vi "TagDB Refmgr-Register.vi"(7 "menu reference":refnum<k9>, 8 "error in (no error)":errorcluster, 9 "ViName":string, 10 "VI Refnum":refnum<vi>, 11 "TagDB in":refnum<k1>) -> (0 "error out":errorcluster, 2 "VI Refnum (dup)":refnum<vi>, 3 "TagDB out":refnum<k1>)   [LabVIEW 2017, in "TagDB RefManager.lvlib"]
uses:
  TagDB RefManager.lvlib
  _Support/Refnum Operation/VI/VIName.vi
  _Support/Refnum Operation/VI/Caller's VI Reference.vi
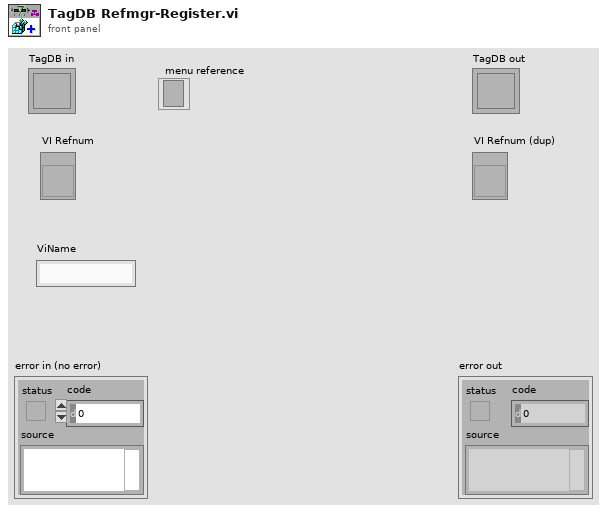
[diagram p1: front panel]
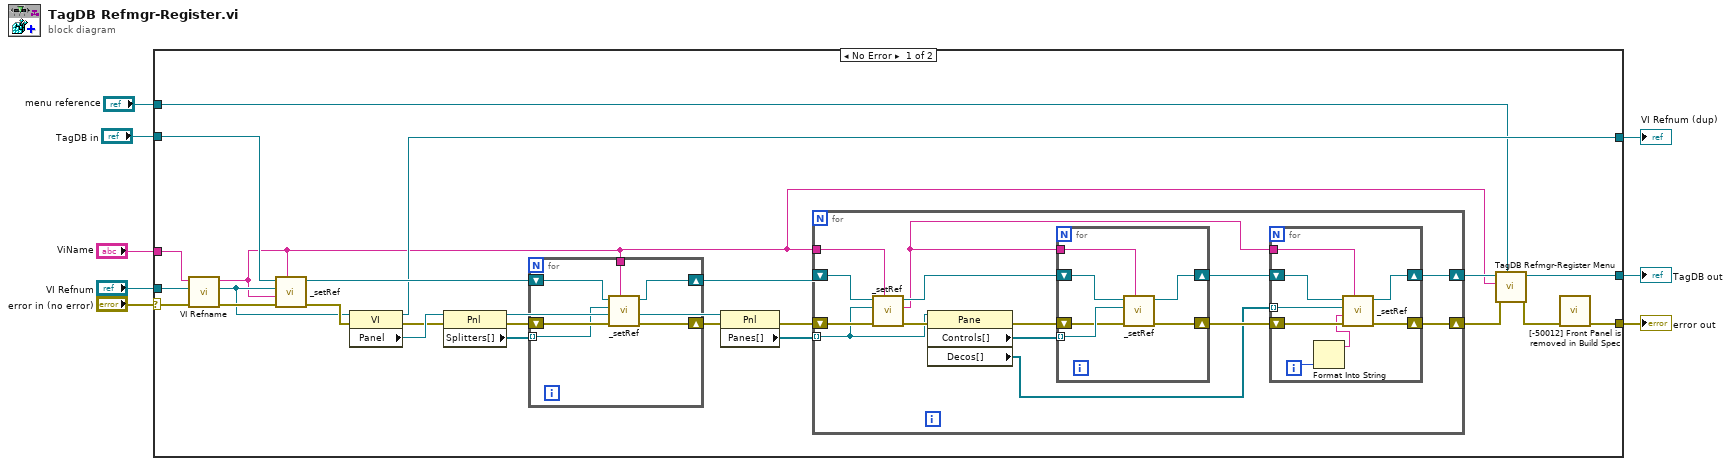
[diagram p0: block diagram]
diagram:
  n1 = case shown="No Error" "error in (no error)" {
    selector: "error in (no error)" -> [w19 w70]
    tunnel: [w18 w70] -> w7
    tunnel: [w11 w69] -> w5
    tunnel: "TagDB in" -> [w21 w69]
    tunnel: "VI Refnum" -> [w16 w68]
    tunnel: "ViName" -> [w17 _]
    tunnel: [w14 w68] -> w2
    tunnel: "menu reference" -> [w10 _]
    frame No Error {
      n2 = call "VI Refname.vi"("error in (no error)"=w19, "VI in"=w16, "ViName"=w17) -> ("error out"=w23:errorcluster, "VI out"=w15:refnum<vi>, "Name"=w9:string)  [unwired: 6 in]
      n3 = call "_setRef.vi"("parentURL"=w9, "error in (no error)"=w23, "Name"=w9, "Refnum"=w15, "TagDB in"=w21) -> ("error out"=w22:errorcluster, "TagDB out"=w20:refnum<k1>)  [unwired: 4 in, 1 out]
      n4 = property class="VI"(reference=w15, error in=w22) -> (reference out=w14:refnum<vi>, error out=w29:errorcluster, "Panel"=w30:refnum<vi>)
      n5 = property class="Pnl"(reference=w30, error in=w29) -> (reference out=w28:refnum<vi>, error out=w26:errorcluster, "Splitters[]"=w25:refnum<vi>[])
      n6 = for {
        shift-right: [w65] -> w27
        shift-left: w20 -> [w66]
        tunnel: w25 -> [w63] mode=indexing
        shift-right: [w64] -> w24
        shift-left: w26 -> [w67]
        tunnel: w9 -> [w62]
        n7 = call "_setRef.vi"("parentURL"=w62, "error in (no error)"=w67, "Refnum"=w63, "TagDB in"=w66) -> ("error out"=w64:errorcluster, "TagDB out"=w65:refnum<k1>)  [unwired: 5 in, 1 out]
      }
      n8 = property class="Pnl"(reference=w28, error in=w24) -> (error out=w31:errorcluster, "Panes[]"=w33:refnum<vi>[])  [unwired: 1 out]
      n9 = for {
        tunnel: w33 -> [w41] mode=indexing
        shift-right: [w37] -> w12
        shift-left: w27 -> [w43]
        shift-right: [w36] -> w32
        shift-left: w31 -> [w45]
        tunnel: w9 -> [w40]
        n10 = call "_setRef.vi"("parentURL"=w40, "error in (no error)"=w45, "Refnum"=w41, "TagDB in"=w43) -> ("error out"=w44:errorcluster, "URL"=w35:string, "TagDB out"=w42:refnum<k1>)  [unwired: 5 in]
        n11 = property class="Pane"(reference=w41, error in=w44) -> (error out=w46:errorcluster, "Controls[]"=w47:refnum<vi>[], "Decos[]"=w34:refnum<vi>[])  [unwired: 1 out]
        n12 = for {
          tunnel: w47 -> [w58] mode=indexing
          shift-right: [w60] -> w38
          shift-left: w42 -> [w61]
          shift-right: [w59] -> w39
          shift-left: w46 -> [w57]
          tunnel: w35 -> [w56]
          n13 = call "_setRef.vi"("parentURL"=w56, "error in (no error)"=w57, "Refnum"=w58, "TagDB in"=w61) -> ("error out"=w59:errorcluster, "TagDB out"=w60:refnum<k1>)  [unwired: 5 in, 1 out]
        }
        n14 = for {
          shift-right: [w54] -> w37
          shift-left: w38 -> [w55]
          shift-right: [w53] -> w36
          shift-left: w39 -> [w52]
          tunnel: w35 -> [w51]
          tunnel: w34 -> [w50] mode=indexing
          i -> [w48]
          n15 = Format Into String(w48) -> (resulting string=w49:string)  [unwired: 3 in, 1 out]
          n16 = call "_setRef.vi"("parentURL"=w51, "error in (no error)"=w52, "Name"=w49, "Refnum"=w50, "TagDB in"=w55) -> ("error out"=w53:errorcluster, "TagDB out"=w54:refnum<k1>)  [unwired: 4 in, 1 out]
        }
      }
      n17 = call "TagDB Refmgr-Register Menu.vi"("menu reference"=w10, "error in (no error)"=w32, "parentURL"=w9, "TagDB in"=w12) -> ("error out"=w13:errorcluster, "TagDB out"=w11:refnum<k1>)  [unwired: 6 in]
      n18 = call "[-50012] Front Panel is removed in Build Spec.vi"("error in (no error)"=w13) -> ("error out"=w18:errorcluster)  [unwired: 10 in]
    }
    frame Error {
    }
  }
  "error out" <- w7
  "TagDB out" <- w5
  "VI Refnum (dup)" <- w2
